vi "Message Based DAQ-solution.vi"() -> ()   [LabVIEW 2014]
uses:
  <vilib>/Utility/error.llb/DialogType.ctl
  vilib/Message/Msg Post UI Message.vi
  <vilib>/DAQmx/create/channels.llb/DAQmx Create Channel (AI-Voltage-Basic).vi
  <vilib>/DAQmx/configure/timing.llb/DAQmx Timing (Sample Clock).vi
  vilib/Message/Msg Post Queue Message.vi
  <vilib>/DAQmx/read.llb/DAQmx Read (Analog Wfm 1Chan NSamp).vi
  vilib/Message/Msg Send Queue Message.vi
  <resource>/objmgr/daqmx.rc
panel:
  in  "File Path":path
  in  "Acquire Data":bool
  in  "Log Data":bool
  in  "File Comment":string
  in  "DAQ Parameters":T1={"physical channels"="", "maximum value"=5.0, "minimum value"=-5.0, "rate"=1000.0, "read period"=0.5} {"read period" format="%0.2f"; "rate" format="%0.2f"; "minimum value" format="%0.2f"; "maximum value" format="%0.2f"}
  out "Waveform Chart":waveform(dbl)(graph)
  in  "quit":bool
  # "V"
  # "V"
  # "Hz"
  # "s"
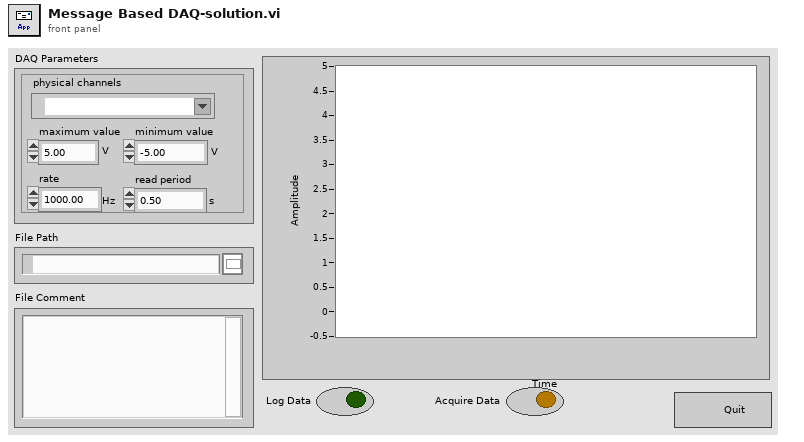
[diagram p1: front panel]
types:
  T1 = cluster{"physical channels":tag, "maximum value":dbl, "minimum value":dbl, "rate":dbl, "read period":dbl}
  T2 = typedef "DialogType.ctl" = u16
  T3 = enum16{"Left Button", "Center Button", "Right Button", "Window Close"}
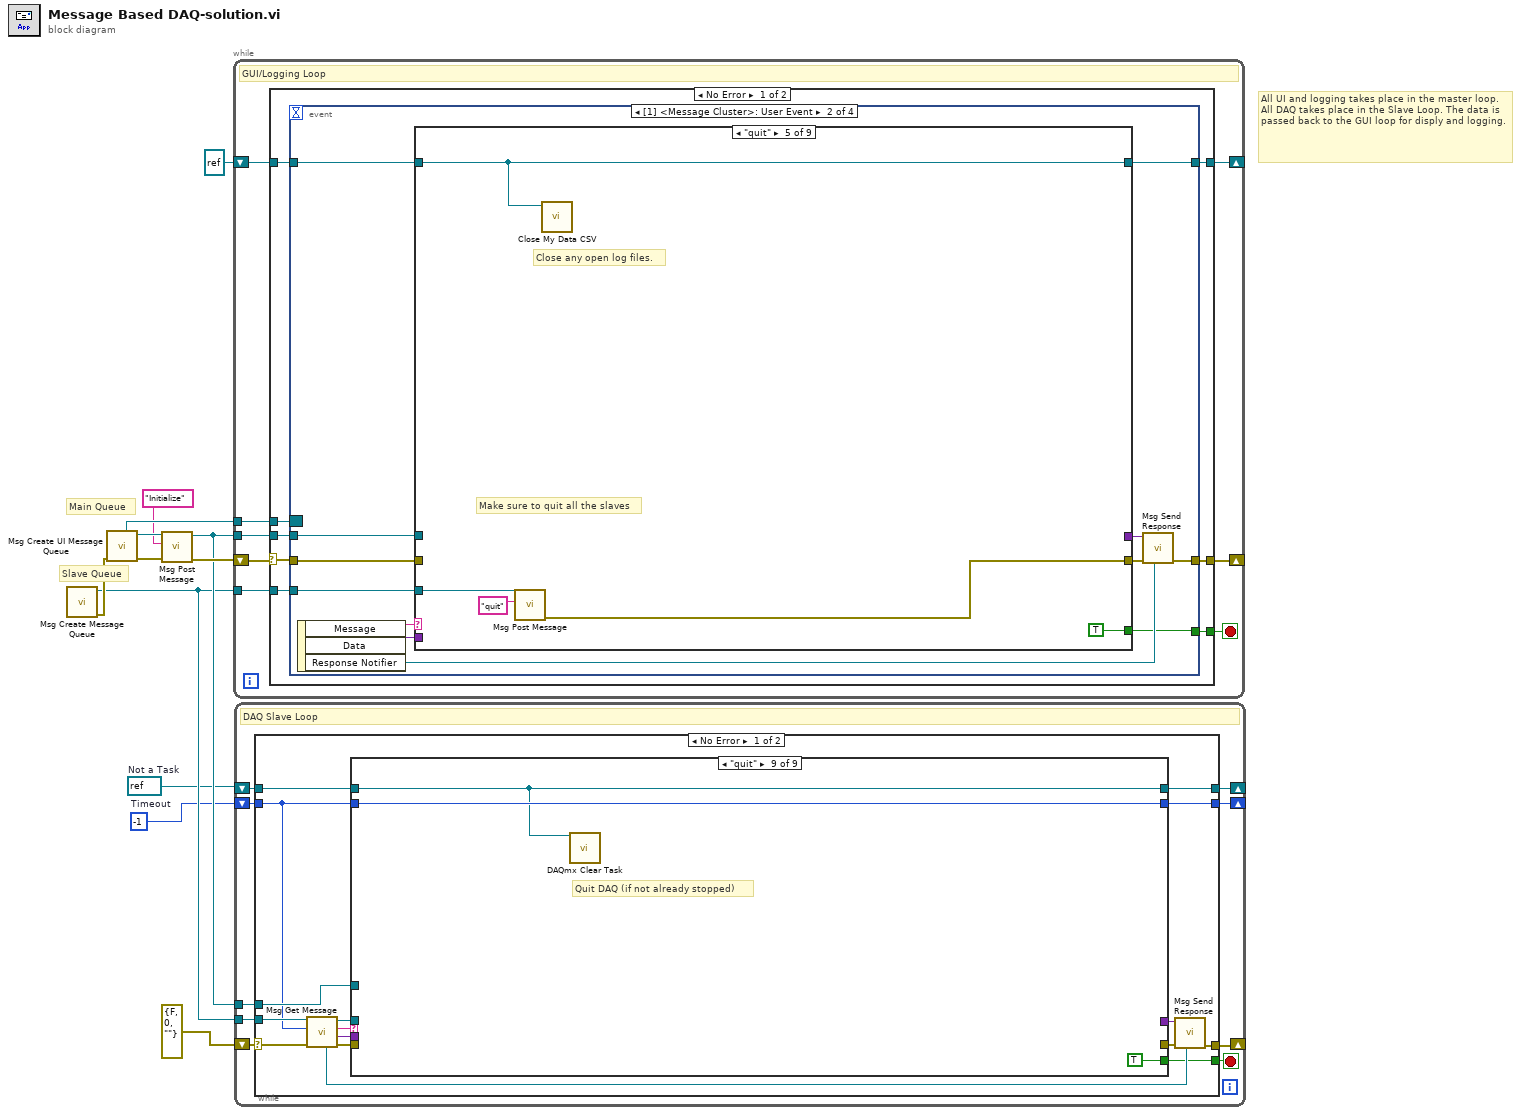
[diagram p0: block diagram]
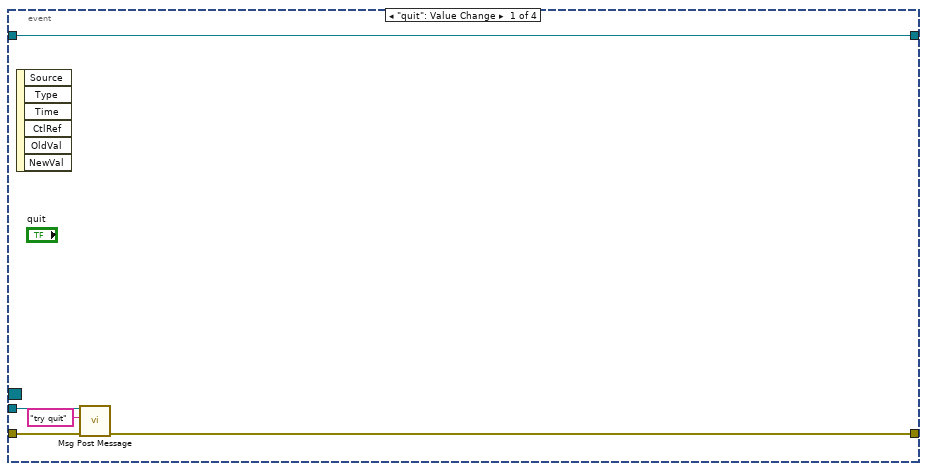
[diagram p2: hidden frame]
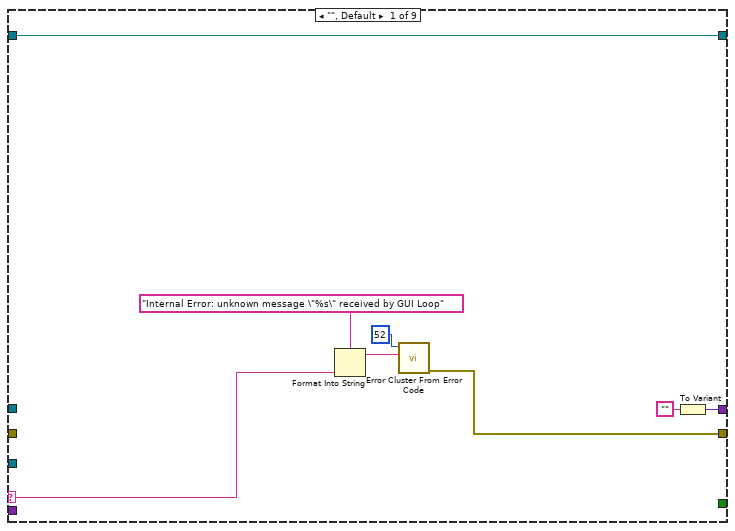
[diagram p3: hidden frame]
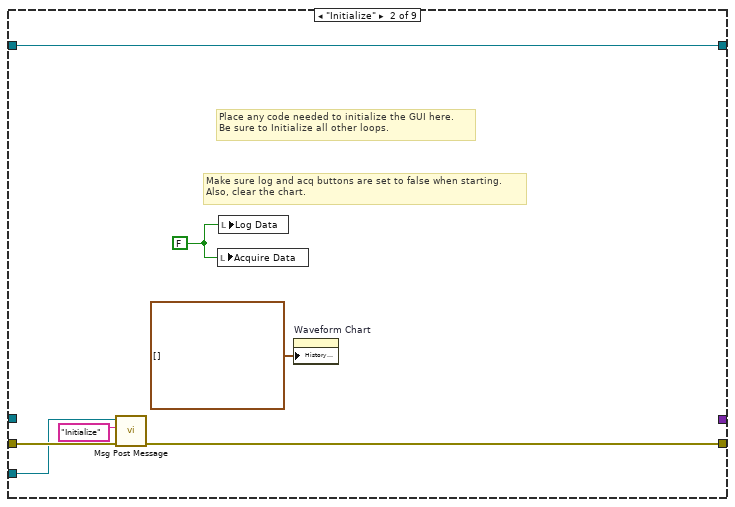
[diagram p4: hidden frame]
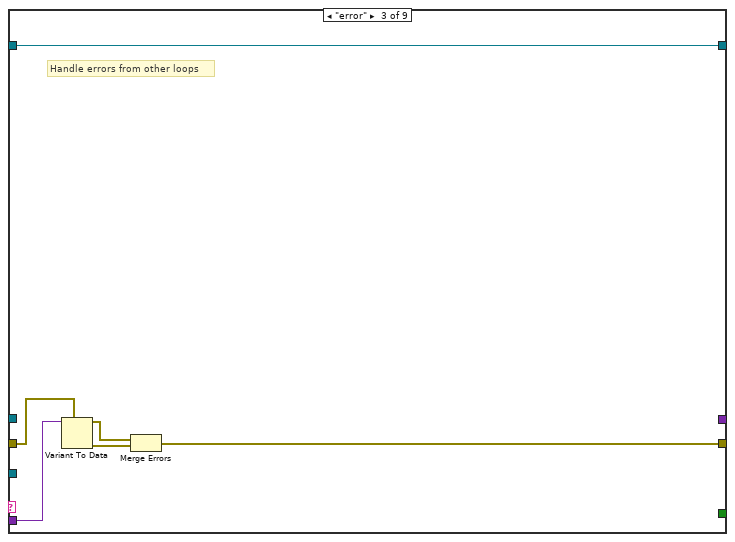
[diagram p5: hidden frame]
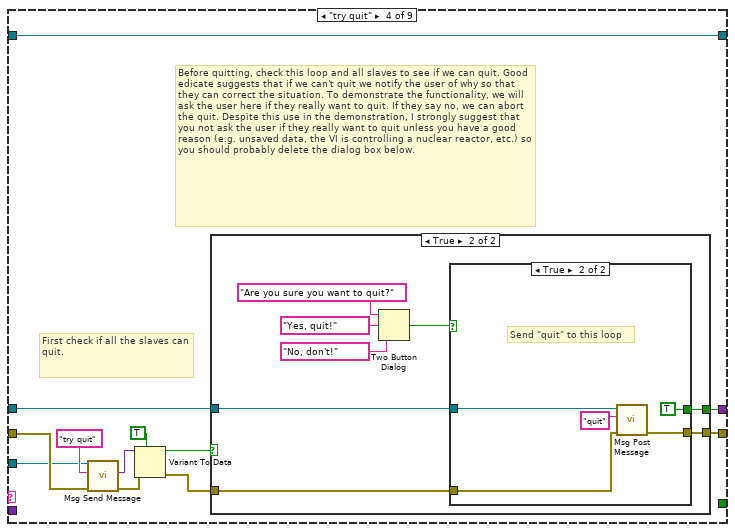
[diagram p6: hidden frame]
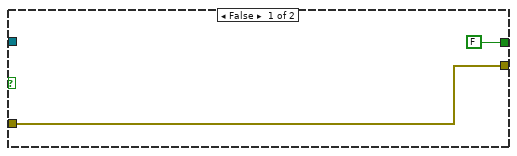
[diagram p7: hidden frame]
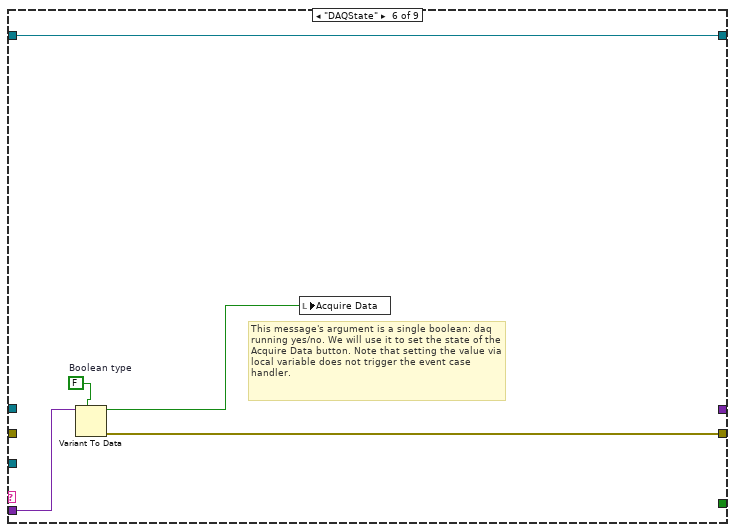
[diagram p9: hidden frame]
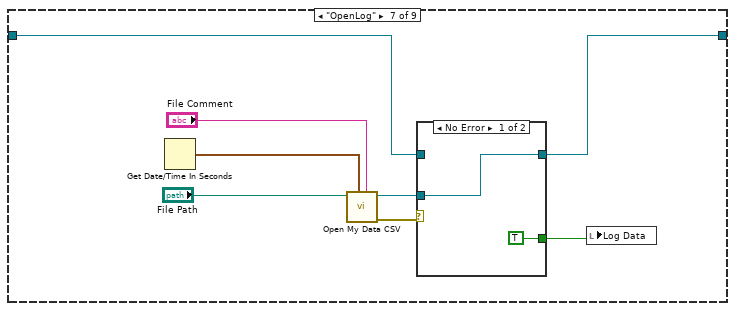
[diagram p10: hidden frame]
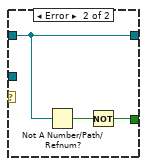
[diagram p11: hidden frame]
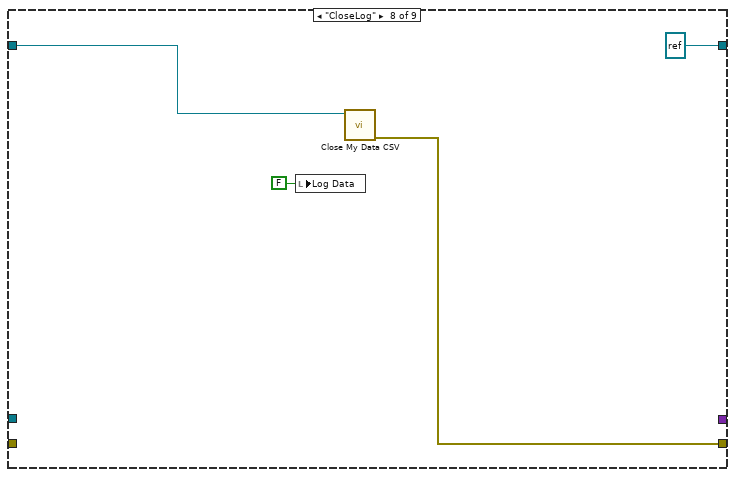
[diagram p12: hidden frame]
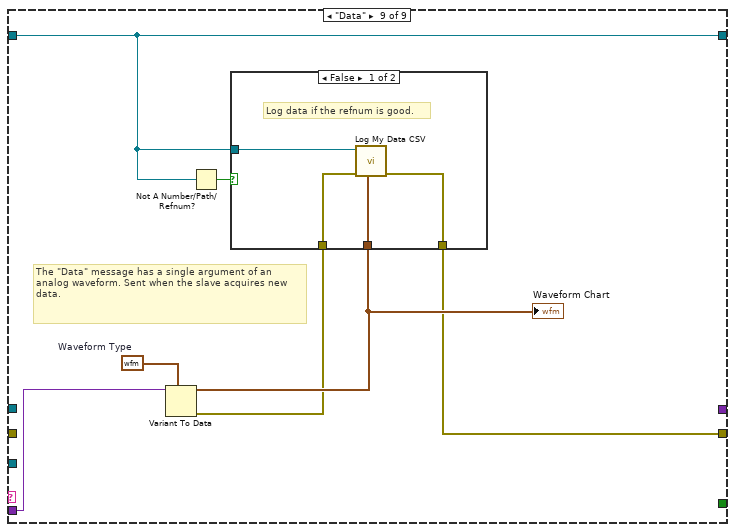
[diagram p13: hidden frame]
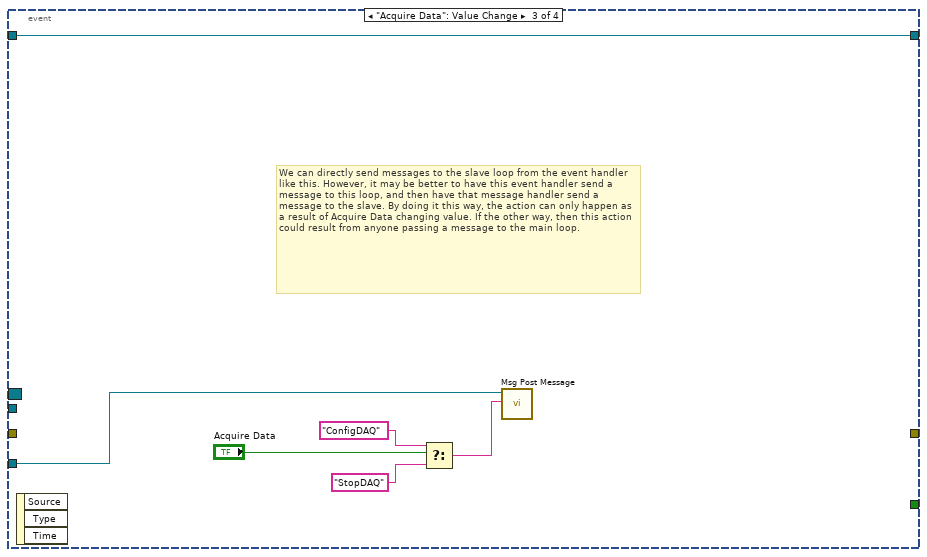
[diagram p15: hidden frame]
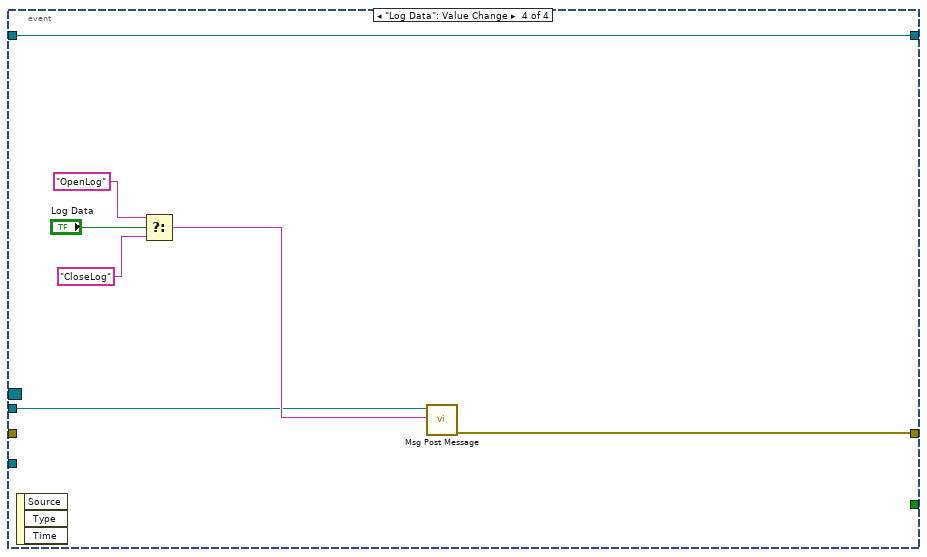
[diagram p16: hidden frame]
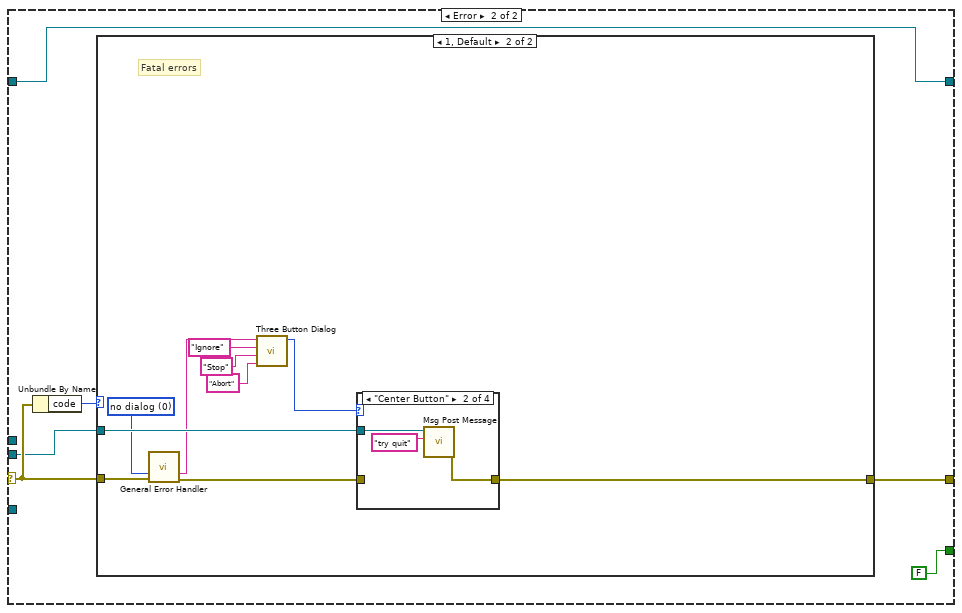
[diagram p17: hidden frame]
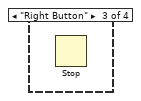
[diagram p20: hidden frame]
diagram:
  w2 = -1  # Timeout
  w3 = refnum<k21> refnum  # Not a Task
  # "All UI and logging takes place in the master loop. All DAQ takes place in the Slave Loop. The data is passed back to the GUI loop for disply and logging."
  # "Main Queue"
  # "Slave Queue"
  n1 = call "Msg Create Message Queue.vi"() -> ("error out"=w8:errorcluster, "queue out"=w5:refnum<queue>)  [unwired: 7 in, 1 out]
  n2 = call "Msg Create UI Message Queue.vi"("error in (no error)"=w8) -> ("error out"=w9:errorcluster, "user event"=w11:refnum<user-event>, "Event Registration Refnum out"=w12:refnum<event-registration>)  [unwired: 6 in]
  n3 = call-poly "Msg Post Message.vi"("error in (no error)"=w9, "Message"="Initialize", "user event"=w11) -> ("error out"=w7:errorcluster, "user event out"=w6:refnum<user-event>)  [unwired: 4 in, 1 out]
  n4 = while {
    tunnel: w12 -> [w19]
    shift-right: [w17] -> _
    shift-left: w7 -> [w15]
    tunnel: w6 -> [w18]
    tunnel: w5 -> [w16]
    shift-right: [w14] -> _
    shift-left: refnum<file> refnum ("refnum out") -> [w13]
    stop <- w20 stop-if-true
    # "GUI/Logging Loop"
    n5 = case shown="No Error" w15 {
      selector: w15 -> [w23 w150]
      tunnel: [w28 FALSE] -> w20
      tunnel: w19 -> [w27 _]
      tunnel: w18 -> [w26 w149]
      tunnel: [w25 w148] -> w17
      tunnel: w16 -> [w24 _]
      tunnel: [w22 w147] -> w14
      tunnel: w13 -> [w21 w147]
      frame No Error {
        n6 = event shown="[1] <Message Cluster>: User Event" {
          selector: w27 -> [_ _ _ _]
          dyn-events: _ -> [_ _ _ _]
          timeout: _ -> [_ _ _ _]
          tunnel: [_ w36 _ _] -> w28
          tunnel: w26 -> [w33 w37 _ w142]
          tunnel: w23 -> [w32 w42 _ _]
          tunnel: [w31 w40 _ w141] -> w25
          tunnel: w24 -> [_ w38 w139 _]
          tunnel: [w29 w35 w134 w140] -> w22
          tunnel: w21 -> [w29 w34 w134 w140]
          event "quit": Value Change {
            n7 = event-data() -> ()  [unwired: 1 in, 6 out]
            n8 = call-poly "Msg Post Message.vi"("error in (no error)"=w32, "Message"="try quit", "user event"=w33) -> ("error out"=w31:errorcluster)  [unwired: 4 in, 2 out]
          }
          event User Event {
            n9 = event-data() -> ("Message"=w45:string, "Data"=w39:variant, "Response Notifier"=w43:refnum<notifier>)  [unwired: 1 in]
            n10 = case shown="\"quit\"" w45 {
              selector: w45 -> [w51 _ _ _ _ _ _ _ _]
              tunnel: [w52 _ _ w71 _ _ _ _ _] -> w44
              tunnel: w42 -> [_ w60 w65 w78 _ _ _ _ _]
              tunnel: [w47 w57 w62 w72 w96 w101 _ w118 w124] -> w41
              tunnel: w39 -> [_ _ w66 _ _ w104 _ _ w128]
              tunnel: w38 -> [_ w59 _ w69 w97 _ _ _ _]
              tunnel: w37 -> [_ _ _ w73 _ _ _ _ _]
              tunnel: [_ _ _ _ TRUE _ _ _ _] -> w36
              tunnel: [w46 w56 w61 w67 w95 w100 w106 refnum<file> refnum ("refnum out") w122] -> w35
              tunnel: w34 -> [w46 w56 w61 w67 w95 w100 w105 w121 w122]
              frame "", Default {
                n11 = Format Into String(format string="Internal Error: unknown message \"%s\" received by GUI Loop" ("error message (\"\")"), w51) -> (resulting string=w48:string)  [unwired: 2 in, 1 out]
                n12 = call <vilib>:"Error Cluster From Error Code.vi"("error message (\"\")"=w48, "error code (0)"=52) -> ("error out"=w47:errorcluster)  [unwired: 7 in]
                n13 = To Variant(anything="") -> (Variant=w52:variant)
              }
              frame "Initialize" {
                w55 = FALSE
                # "Make sure log and acq buttons are set to false when starting.\nAlso, clear the chart."
                # "Place any code needed to initialize the GUI here. \nBe sure to Initialize all other loops."
                n14 = call-poly "Msg Post Message.vi"("error in (no error)"=w60, "Message"="Initialize", "queue"=w59) -> ("error out"=w57:errorcluster)  [unwired: 4 in, 2 out]
                n15 = local write "Acquire Data"(w55) -> ()
                n16 = local write "Log Data"(w55) -> ()
                n17 = property on="Waveform Chart" class="WFChart (strict)"("History Data"=waveform(dbl)[] []) -> ()  [unwired: 2 in, 2 out]
              }
              frame "error" {
                # "Handle errors from other loops"
                n18 = Variant To Data(type=w65, Variant=w66) -> (data=w64:errorcluster, error out=w63:errorcluster)  [unwired: 1 in]
                n19 = Merge Errors(w64, w63) -> (w62:errorcluster)
              }
              frame "try quit" {
                # "Before quitting, check this loop and all slaves to see if we can quit. Good edicate suggests that if we can't quit we notify the user of why so that they can correct the situation. To demonstrate the functionality, we will ask the user here if they really want to quit. If they say no, we can abort the quit. Despite this use in the demonstration, I strongly suggest that you not ask the user if they really want to quit unless you have a good reason (e.g. unsaved data, the VI is controlling a nuclear reactor, etc.) so you should probably delete the dialog box below."
                # "First check if all the slaves can quit."
                n20 = call-poly "Msg Send Message.vi"("error in (no error)"=w78, "Message"="try quit", "queue"=w69) -> ("error out"=w76:errorcluster, "response"=w70:variant)  [unwired: 3 in, 2 out]
                n21 = Variant To Data(error in=w76, type=TRUE, Variant=w70) -> (data=w68:bool, error out=w74:errorcluster)
                n22 = case shown="True" w68 {
                  tunnel: w74 -> [w80 w87]
                  tunnel: w73 -> [_ w88]
                  tunnel: [w80 w86] -> w72
                  tunnel: [FALSE w85] -> w71
                  frame False {
                  }
                  frame True {
                    n23 = Two Button Dialog(message="Are you sure you want to quit?", 1:"No, don't!" ("T button name (\"OK\")"), 2:"Yes, quit!" ("T button name (\"OK\")")) -> (T button?=w81:bool)
                    n24 = case shown="True" w81 {
                      tunnel: w88 -> [_ w94]
                      tunnel: w87 -> [w89 w92]
                      tunnel: [w89 w91] -> w86
                      tunnel: [_ TRUE] -> w85
                      frame False {
                      }
                      frame True {
                        # "Send \"quit\" to this loop"
                        n25 = call-poly "Msg Post Message.vi"("error in (no error)"=w92, "Message"="quit", "user event"=w94) -> ("error out"=w91:errorcluster)  [unwired: 4 in, 2 out]
                      }
                    }
                  }
                }
              }
              frame "quit" {
                # "Close any open log files."
                # "Make sure to quit all the slaves"
                n26 = call-poly "Msg Post Message.vi"("Message"="quit", "queue"=w97) -> ("error out"=w96:errorcluster)  [unwired: 5 in, 2 out]
                n27 = call "Close My Data CSV.vi"("file refnum"=w95) -> ()  [unwired: 10 in, 1 out]
              }
              frame "DAQState" {
                w103 = FALSE  # Boolean type
                # "This message's argument is a single boolean: daq running yes/no. We will use it to set the state of the Acquire Data button. Note that setting the value via local variable does not trigger the event case handler."
                n28 = Variant To Data(type=w103, Variant=w104) -> (data=w102:bool, error out=w101:errorcluster)  [unwired: 1 in]
                n29 = local write "Acquire Data"(w102) -> ()
              }
              frame "OpenLog" {
                n30 = Get Date/Time In Seconds() -> (seconds since 1Jan1904=w110:timestamp)
                n31 = call "Open My Data CSV.vi"("Comment"="File Comment", "Time Stamp"=w110, "file path"="File Path") -> ("error out"=w109:errorcluster, "refnum out"=w107:refnum<file>)  [unwired: 7 in]
                n32 = case shown="No Error" w109 {
                  tunnel: [TRUE w116] -> w108
                  tunnel: w107 -> [w113 _]
                  tunnel: [w113 w117] -> w106
                  tunnel: w105 -> [_ w117]
                  frame No Error {
                  }
                  frame Error {
                    n33 = Not A Number/Path/Refnum?(number/path/refnum=w117) -> (NaN/Path/Refnum?=w115:bool)
                    n34 = Not(x=w115) -> (.not. x?=w116:bool)
                  }
                }
                n35 = local write "Log Data"(w108) -> ()
              }
              frame "CloseLog" {
                n36 = local write "Log Data"(FALSE ("Log Data")) -> ()
                n37 = call "Close My Data CSV.vi"("file refnum"=w121) -> ("error out"=w118:errorcluster)  [unwired: 10 in]
              }
              frame "Data" {
                w127 = waveform(dbl) {"t0"=timestamp(0 s since 1904-01-01), "dt"=1.0, "Y"=[]}  # Waveform Type
                # "The \"Data\" message has a single argument of an analog waveform. Sent when the slave acquires new data."
                n38 = Variant To Data(type=w127, Variant=w128) -> (data=w126:waveform(dbl), error out=w125:errorcluster)  [unwired: 1 in]
                "Waveform Chart" <- w126
                n39 = Not A Number/Path/Refnum?(number/path/refnum=w122) -> (NaN/Path/Refnum?=w123:bool)
                n40 = case shown="False" w123 {
                  tunnel: w126 -> [w132 _]
                  tunnel: w125 -> [w131 w133]
                  tunnel: [w130 w133] -> w124
                  tunnel: w122 -> [w129 _]
                  frame False {
                    # "Log data if the refnum is good."
                    n41 = call "Log My Data CSV.vi"("Data"=w132, "error in"=w131, "file refnum"=w129) -> ("error out"=w130:errorcluster)  [unwired: 7 in, 1 out]
                  }
                  frame True {
                  }
                }
              }
            }
            n42 = call "Msg Send Response.vi"("Response Notifier"=w43, "error in (no error)"=w41, "response"=w44) -> ("error out"=w40:errorcluster)  [unwired: 6 in]
          }
          event "Acquire Data": Value Change {
            # "We can directly send messages to the slave loop from the event handler like this. However, it may be better to have this event handler send a message to this loop, and then have that message handler send a message to the slave. By doing it this way, the action can only happen as a result of Acquire Data changing value. If the other way, then this action could result from anyone passing a message to the main loop."
            n43 = event-data() -> ()  [unwired: 1 in, 3 out]
            n44 = Select(t="ConfigDAQ" ("Message"), s="Acquire Data", f="StopDAQ" ("Message")) -> (s? t:f=w135:string)
            n45 = call-poly "Msg Post Message.vi"("Message"=w135, "queue"=w139) -> ()  [unwired: 5 in, 3 out]
          }
          event "Log Data": Value Change {
            n46 = event-data() -> ()  [unwired: 1 in, 3 out]
            n47 = Select(t="OpenLog" ("Message"), s="Log Data", f="CloseLog" ("Message")) -> (s? t:f=w143:string)
            n48 = call-poly "Msg Post Message.vi"("Message"=w143, "user event"=w142) -> ("error out"=w141:errorcluster)  [unwired: 5 in, 2 out]
          }
        }
      }
      frame Error {
        n49 = Unbundle By Name(w150) -> ("code"=w151:i32)
        n50 = case shown="1, Default" w151 {
          tunnel: w150 -> [_ w162]
          tunnel: w149 -> [_ w161]
          tunnel: [_ w159] -> w148
          frame 0 {
            # "Ignore these errors"
          }
          frame 1, Default {
            w158 = T2 0 items=["no dialog", "OK message", "continue or stop message", "OK message + warnings", "continue/stop + warnings"] ("type of dialog (OK msg:1)")
            # "Fatal errors"
            n51 = call <vilib>:"General Error Handler.vi"("type of dialog (OK msg:1)"=w158, "error in (no error)"=w162) -> ("message"=w157:string, "error out"=w160:errorcluster)  [unwired: 9 in, 3 out]
            n52 = call <vilib>:"Three Button Dialog.vi"("Right Button Text (\"Cancel\")"="Abort" ("Right Button Text (\"Cancel\")"), "Center Button Text (\"No\")"="Stop" ("Center Button Text (\"No\")"), "Left Button Text (\"Yes\")"="Ignore" ("Left Button Text (\"Yes\")"), "message"=w157) -> ("Which Button?"=w153:T3)  [unwired: 7 in]
            n53 = case shown="\"Center Button\"" w153 {
              tunnel: w161 -> [_ w165 _ _]
              tunnel: w160 -> [_ _ _ _]
              tunnel: [_ w163 _ _] -> w159
              frame "Left Button", Default {
              }
              frame "Center Button" {
                n54 = call-poly "Msg Post Message.vi"("Message"="try quit", "user event"=w165) -> ("error out"=w163:errorcluster)  [unwired: 5 in, 2 out]
              }
              frame "Right Button" {
                n55 = Stop() -> ()  [unwired: 1 in]
              }
              frame "Window Close" {
              }
            }
          }
        }
      }
    }
  }
  n56 = while {
    tunnel: w6 -> [w170]
    tunnel: w5 -> [w174]
    shift-right: [w173] -> _
    shift-left: errorcluster {"status"=FALSE, "code"=0, "source"=""} ("error out") -> [w171]
    shift-right: [w169] -> _
    shift-left: w3 -> [w168]
    shift-right: [w167] -> _
    shift-left: w2 -> [w166]
    stop <- w172 stop-if-true
    # "DAQ Slave Loop"
    n57 = case shown="No Error" w171 {
      selector: w171 -> [w180 w283]
      tunnel: w174 -> [w190 _]
      tunnel: [w184 w282] -> w173
      tunnel: [w181 _] -> w172
      tunnel: w170 -> [w177 w285]
      tunnel: [w179 w281] -> w169
      tunnel: w168 -> [w178 w281]
      tunnel: [w176 w280] -> w167
      tunnel: w166 -> [w175 w280]
      frame No Error {
        n58 = call "Msg Get Message.vi"("queue"=w190, "timeout in ms (-1)"=w175, "error in (no error)"=w180) -> ("Response Notifier"=w183:refnum<notifier>, "queue out"=w186:refnum<queue>, "Message"=w188:string, "Data"=w187:variant, "error out"=w189:errorcluster)  [unwired: 1 in]
        n59 = case shown="\"quit\"" w188 {
          selector: w188 -> [w193 _ _ _ _ _ _ _ _]
          tunnel: [w194 _ w208 w232 w254 w259 w268 _ _] -> w185
          tunnel: w189 -> [_ _ _ _ _ _ _ _ _]
          tunnel: w187 -> [_ _ _ _ _ _ _ _ _]
          tunnel: w186 -> [_ _ w209 _ w257 _ _ _ _]
          tunnel: [w199 _ _ _ _ _ _ TRUE _] -> w182
          tunnel: [FALSE _ _ _ _ _ _ _ TRUE] -> w181
          tunnel: [w192 w202 w206 w240 w258 w263 w272 w274 w277] -> w179
          tunnel: w178 -> [w192 w202 w203 w240 w258 w265 w272 w274 w277]
          tunnel: w177 -> [_ _ _ w231 _ w261 w270 _ _]
          tunnel: [w191 w201 w205 w235 -1 w262 w273 w275 w278] -> w176
          tunnel: w175 -> [w191 w201 w204 w234 _ w262 w273 w275 w278]
          frame "", Default {
            n60 = Format Into String(format string="Internal Error: unknown message \"%s\" received by Slave Loop 1" ("error message (\"\")"), w193) -> (resulting string=w197:string)  [unwired: 2 in, 1 out]
            n61 = call <vilib>:"Error Cluster From Error Code.vi"("error message (\"\")"=w197, "error code (0)"=52) -> ("error out"=w194:errorcluster)  [unwired: 7 in]
            n62 = To Variant(anything="") -> (Variant=w199:variant)
          }
          frame "Initialize" {
          }
          frame "ConfigDAQ" {
            w215 = 10123 items=["Finite Samples"=10178, "Continuous Samples"=10123, "Hardware Timed Single Point"=12522] ("sample mode")
            n63 = Unbundle By Name("DAQ Parameters") -> ("read period"=w212:dbl, "rate"=w214:dbl, "minimum value"=w218:dbl, "maximum value"=w217:dbl, "physical channels"=w219:tag)
            n64 = call-poly <vilib>:"DAQmx Create Virtual Channel.vi"("maximum value"=w217, "minimum value"=w218, "physical channels"=w219) -> ("task out"=w211:refnum<k21>, "error out"=w216:errorcluster)  [unwired: 11 in]
            n65 = Multiply(x=w212, y=w214) -> (x*y=w213:dbl)
            n66 = call-poly <vilib>:"DAQmx Timing.vi"("task/channels in"=w211, "sample mode"=w215, "samples per channel"=w213, "rate"=w214, "error in"=w216) -> ("task out"=w207:refnum<k21>, "error out"=w210:errorcluster)  [unwired: 9 in]
            n67 = case shown="No Error" w210 {
              selector: w210 -> [w224 w227]
              tunnel: w209 -> [w225 _]
              tunnel: [w223 w227] -> w208
              tunnel: w207 -> [w222 _]
              tunnel: [w222 w228] -> w206
              tunnel: [w221 w229] -> w205
              tunnel: w204 -> [w221 w229]
              tunnel: w203 -> [_ w228]
              frame No Error {
                n68 = call-poly "Msg Post Message.vi"("error in (no error)"=w224, "Message"="StartDAQ", "queue"=w225) -> ("error out"=w223:errorcluster)  [unwired: 4 in, 2 out]
              }
              frame Error {
              }
            }
          }
          frame "StartDAQ" {
            # "Notify master of change in DAQ state"
            n69 = property class="DAQmx Timing"(reference=w240) -> (reference out=w236:refnum<k21>, error out=w237:errorcluster, "SampQuant.SampPerChan"=w239:dbl, "SampClk.Rate"=w238:dbl)  [unwired: 1 in]
            n70 = call <vilib>:"DAQmx Start Task.vi"("task/channels in"=w236, "error in"=w237) -> ("error out"=w241:errorcluster)  [unwired: 12 in, 1 out]
            n71 = case shown="No Error" w241 {
              selector: w241 -> [w246 w253]
              tunnel: w239 -> [w249 _]
              tunnel: w238 -> [w248 _]
              tunnel: [w247 w252] -> w235
              tunnel: w234 -> [_ w252]
              tunnel: [w246 w253] -> w232
              tunnel: [TRUE w250] -> w230
              frame No Error {
                n72 = Divide(x=w249, y=w248) -> (x/y=w244:dbl)
                n73 = Multiply(x=1000.0 ("y"), y=w244) -> (x*y=w242:dbl)
                n74 = To Long Integer(number=w242) -> (32bit integer=w247:i32)
              }
              frame Error {
                n75 = Not Equal?(x=w252, y=-1) -> (x != y?=w250:bool)
              }
            }
            n76 = call-poly "Msg Post Message.vi"("Data"=w230, "Message"="DAQState", "user event"=w231) -> ()  [unwired: 4 in, 3 out]
          }
          frame "StopDAQ" {
            n77 = call <vilib>:"DAQmx Stop Task.vi"("task/channels in"=w258) -> ("error out"=w254:errorcluster)  [unwired: 13 in, 1 out]
            n78 = call-poly "Msg Post Message.vi"("Message"="ClearDAQ", "queue"=w257) -> ()  [unwired: 5 in, 3 out]
          }
          frame "ClearDAQ" {
            w263 = refnum<k21> refnum  # Not a Task
            # "Notify master that DAQ is done."
            n79 = call <vilib>:"DAQmx Clear Task.vi"("task in"=w265) -> ("error out"=w259:errorcluster)  [unwired: 14 in]
            n80 = call-poly "Msg Post Message.vi"("Data"=FALSE, "Message"="DAQState", "user event"=w261) -> ()  [unwired: 4 in, 3 out]
          }
          frame "timeout" {
            # "Read data on timeout.\nPost the data back to the main loop for display and logging.\nThese things could also be done in this loop, but posting it\nback to the main loop allows the slave to operate as efficiently\nas possible."
            n81 = call-poly <vilib>:"DAQmx Read.vi"("task/channels in"=w272, "number of samples per channel"=-1) -> ("data"=w266:waveform(dbl), "error out"=w269:errorcluster)  [unwired: 11 in, 1 out]
            n82 = call-poly "Msg Post Message.vi"("error in (no error)"=w269, "Data"=w266, "Message"="Data", "user event"=w270) -> ("error out"=w268:errorcluster)  [unwired: 3 in, 2 out]
          }
          frame "try quit" {
            # "Perform any preparation for quitting here. This message is sent (not posted) by the main loop. If you are unable to quit, return False, otherwise return True."
          }
          frame "quit" {
            # "Quit DAQ (if not already stopped)"
            n83 = call <vilib>:"DAQmx Clear Task.vi"("task in"=w277) -> ()  [unwired: 14 in, 1 out]
          }
        }
        n84 = call "Msg Send Response.vi"("Response Notifier"=w183, "error in (no error)"=w185, "response"=w182) -> ("error out"=w184:errorcluster)  [unwired: 6 in]
      }
      frame Error {
        # "By default, send errors to the main loop for handling."
        n85 = call-poly "Msg Post Message.vi"("Data"=w283, "Message"="error", "user event"=w285) -> ("error out"=w282:errorcluster)  [unwired: 4 in, 2 out]
      }
    }
  }
